vi "PicoScope Test.vi"(2 "WFD-Ref Ch-B":refnum<vi>, 3 "WFD-Ref Ch-A":refnum<vi>, 8 "Acquisition Settings":T3={"preTriggerSamples"=0, "postTriggerSamples"=1000, "timebase"=127, "Down-Sample Mode"=0, "Down Sample Ratio"=1, "Oversample"=0} {"Down Sample Ratio" min=1 step=1; "Down-Sample Mode" items=["None"=0, "Aggregate"=1, "Decimate"=2, "Average"=4]; "postTriggerSamples" max=10000 step=100}, 9 "Trigger Settings":T4={"Trigger Enabled"=FALSE, "Trigger Source"=enum."Channel A", "Trigger Threshold (Volts)"=0.0, "Trigger Direction"=2, "Trigger Delay (samples)"=0, "Auto Trigger Time (ms)"=1000} {"Trigger Direction" items=["Rising"=2, "Falling"=3]}, 10 "Channel B Settings":T1={"Enabled"=TRUE, "Coupling"=1, "Range"=6, "Analogue Offset"=0.0} {"Range" items=["20 mV"=1, "50 mV"=2, "100 mV"=3, "200 mV"=4, "500 mV"=5, "1 V"=6, "2 V"=7, "5 V"=8, "10 V"=9, "20 V"=10]; "Coupling" items=["AC", "DC"]}, 11 "Channel A Settings":T1={"Enabled"=TRUE, "Coupling"=1, "Range"=6, "Analogue Offset"=0.0} {"Range" items=["20 mV"=1, "50 mV"=2, "100 mV"=3, "200 mV"=4, "500 mV"=5, "1 V"=6, "2 V"=7, "5 V"=8, "10 V"=9, "20 V"=10]; "Coupling" items=["AC", "DC"]}) -> (0 "error out":errorcluster, 5 "Properties Panel":T2 {"Max Total Capture Time Available (sec)" format="%.3p"; "Sample Frequency" format="%.3p"; "Sample Internal" format="%.3p"; "Max Samples Available" format="%.3p"; "Total Capture Time (sec)" format="%.3p"})   [LabVIEW 2018]
panel:
  out "Channel B":cluster{i32, "Sample Internal":sgl, dbl[]}(graph)
  out "Peak To Peak":dbl
  out "Channel A":cluster{i32, "Sample Internal":sgl, dbl[]}(graph)
  out "Serial":string
  out "PicoScope Type":string
  # "Dev Info"
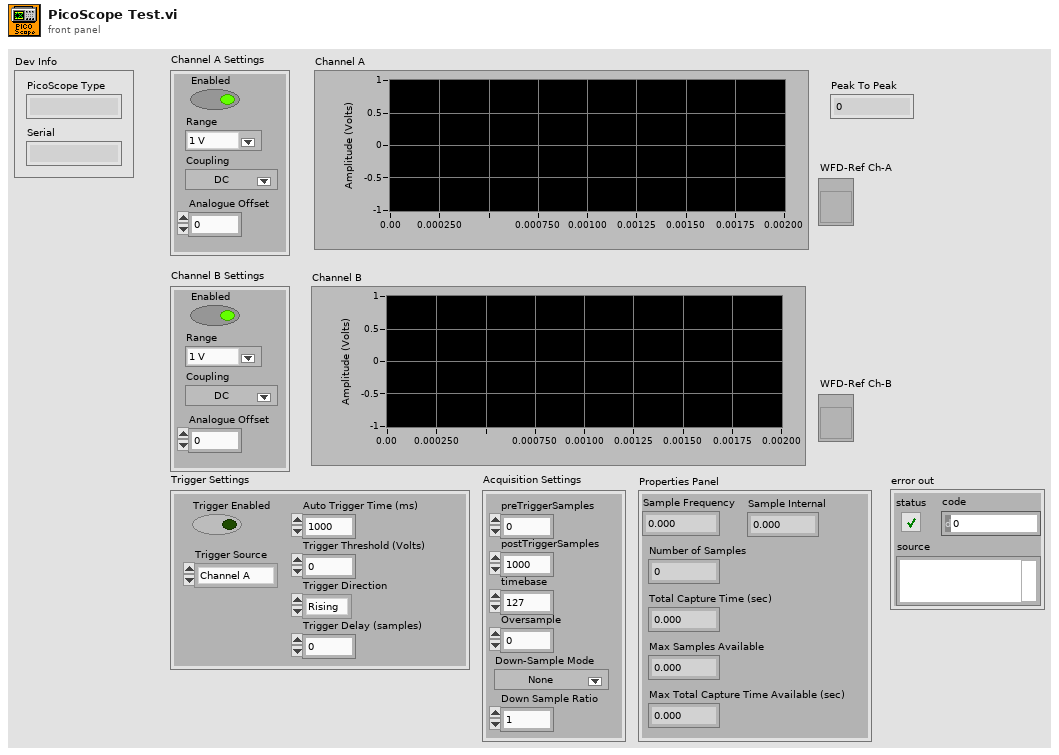
[diagram p1: front panel]
types:
  T1 = cluster{"Enabled":bool, "Coupling":i16, "Range":u16, "Analogue Offset":sgl}
  T2 = cluster{"Sample Frequency":sgl, "Sample Internal":sgl, "Max Samples Available":i32, "Number of Samples":u32, "Total Capture Time (sec) ":sgl, "Max Total Capture Time Available (sec)":sgl}
  T3 = cluster{"preTriggerSamples":u32, "postTriggerSamples":u32, "timebase":u32, "Down-Sample Mode":i32, "Down Sample Ratio":u32, "Oversample":i16}
  T4 = cluster{"Trigger Enabled":bool, "Trigger Source":enum16{"Channel A", "Channel B", "Channel C", "Channel D", "Ext."}, "Trigger Threshold (Volts)":dbl, "Trigger Direction":u16, "Trigger Delay (samples)":u32, "Auto Trigger Time (ms)":i16}
  T5 = cluster{"Driver Version":string, "USB Version":string, "Hardware":string, "Variant":string, "Batch and Serial":string, "Cal Date":string, "Kernel Version":string, "Digital HW Version":string, "Analogue HW Version":string, "Firmware 1":string, "Firmware 2":string, "MSO":bool, "Number of Channels":i16}
  T6 = cluster{"Channel D Buffer":i16[], "Channel C Buffer":i16[], "Channel B Buffer":i16[], "Channel A Buffer":i16[], "Port 0  Buffer ":i16[], "Port 1 Buffer ":i16[]}
  T7 = cluster{i32, "Sample Internal":sgl, "Data (Volts)":dbl[]}
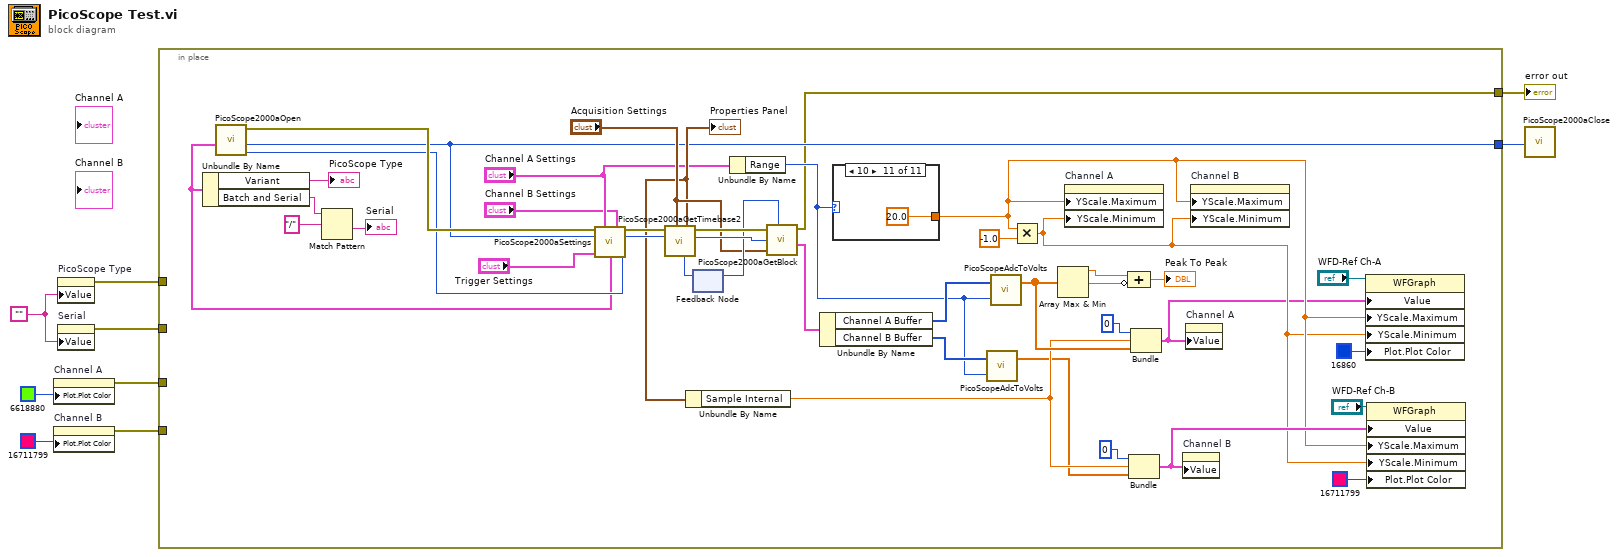
[diagram p0: block diagram]
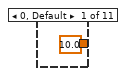
[diagram p2: hidden frame]
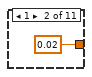
[diagram p3: hidden frame]
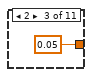
[diagram p4: hidden frame]
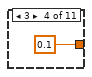
[diagram p5: hidden frame]
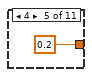
[diagram p6: hidden frame]
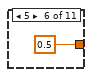
[diagram p7: hidden frame]
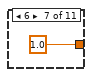
[diagram p8: hidden frame]
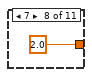
[diagram p9: hidden frame]
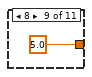
[diagram p10: hidden frame]
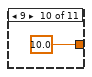
[diagram p11: hidden frame]
diagram:
  w7 = ""
  n1 = property on="Channel A" class="WFGraph (strict)"("Plot.Plot Color"=u32 6618880) -> (error out=w4:errorcluster)  [unwired: 2 in, 1 out]
  n2 = property on="Channel B" class="WFGraph (strict)"("Plot.Plot Color"=u32 16711799) -> (error out=w3:errorcluster)  [unwired: 2 in, 1 out]
  n3 = property on="PicoScope Type" class="Str"("Value"=w7) -> (error out=w9:errorcluster)  [unwired: 2 in, 1 out]
  n4 = property on="Serial" class="Str"("Value"=w7) -> (error out=w8:errorcluster)  [unwired: 2 in, 1 out]
  n5 = in-place {
    in-place-border: w9 -> [_]
    in-place-border: w8 -> [_]
    in-place-border: w4 -> [_]
    in-place-border: w3 -> [_]
    in-place-border: [w14] -> w2
    in-place-border: [w13] -> w1
    n6 = call "PicoScope2000aOpen.vi"() -> ("Max Adc value"=w45:i16, "handle"=w14:i16, "error out"=w46:errorcluster, "Device Info"=w44:T5)  [unwired: 4 in]
    n7 = Unbundle By Name(w44) -> ("Variant"=→"PicoScope Type":string, "Batch and Serial"=w49:string)
    n8 = Match Pattern(string=w49, regular expression="/") -> (after substring=→"Serial":string)  [unwired: 1 in, 3 out]
    n9 = call "PicoScope2000aSettings.vi"("error in"=w46, "Channel A Settings"="Channel A Settings", "Channel B Settings"="Channel B Settings", "handle in"=w14, "Trigger Settings"="Trigger Settings", "Device Info"=w44, "Max_adc"=w45) -> ("error out"=w42:errorcluster, "handle out"=w41:i16)  [unwired: 6 in, 1 out]
    n10 = feedback #1() -> (w37:u32)  [unwired: 1 in]
    n11 = call "PicoScope2000aGetTimebase2.vi"("Number of Samples"=w37, "Acquisition Settings"="Acquisition Settings", "handle in"=w41, "error in (no error)"=w42) -> ("handle out"=w39:i16, "error out"=w40:errorcluster, "Properties Panel"=w33:T2)  [unwired: 5 in]
    "Properties Panel" <- w33
    n12 = Unbundle By Name(w33) -> ("Sample Internal"=w21:sgl)
    n13 = Unbundle By Name("Channel A Settings") -> ("Range"=w23:u16)
    n14 = call "PicoScope2000aGetBlock.vi"("error in"=w40, "handle in"=w39, "Acquisition Settings"="Acquisition Settings") -> ("noOfSamples"=w38:u32, "error out"=w13:errorcluster, "Buffers (Max or non-aggregated)"=w35:T6)  [unwired: 2 in, 3 out]
    n15 = feedback-in #1(w38) -> ()
    n16 = Unbundle By Name(w35) -> ("Channel A Buffer"=w32:i16[], "Channel B Buffer"=w24:i16[])
    n17 = case shown="10" w23 {
      tunnel: [10.0 0.02 0.05 0.1 0.2 0.5 1.0 2.0 5.0 10.0 20.0] -> w16
      frame 0, Default {
      }
      frame 1 {
      }
      frame 2 {
      }
      frame 3 {
      }
      frame 4 {
      }
      frame 5 {
      }
      frame 6 {
      }
      frame 7 {
      }
      frame 8 {
      }
      frame 9 {
      }
      frame 10 {
      }
    }
    n18 = call "PicoScopeAdcToVolts.vi"("Range Index"=w23, "Data"=w24) -> ("Data (Volts)"=w20:dbl[])  [unwired: 1 in]
    n19 = call "PicoScopeAdcToVolts.vi"("Range Index"=w23, "Data"=w32) -> ("Data (Volts)"=w30:dbl[])  [unwired: 1 in]
    n20 = Multiply(x=w16, y=-1.0) -> (x*y=w15:dbl)
    n21 = Array Max & Min(array=w30) -> (max value=w28:dbl, min value=w26:dbl)  [unwired: 2 out]
    n22 = property on="Channel A" class="WFGraph (strict)"("YScale.Maximum"=w16, "YScale.Minimum"=w15) -> ()  [unwired: 2 in, 2 out]
    n23 = Compound Arithmetic op=ADD(w28, invert w26) -> (→"Peak To Peak":dbl)
    n24 = Bundle(0, "Sample Internal"=w21, "Data (Volts)"=w20) -> (w18:T7)  [unwired: 1 in]
    n25 = Bundle(0, "Sample Internal"=w21, "Data (Volts)"=w30) -> (w12:T7)  [unwired: 1 in]
    n26 = property on="Channel B" class="WFGraph (strict)"("Value"=w18) -> ()  [unwired: 2 in, 2 out]
    n27 = property on="Channel A" class="WFGraph (strict)"("Value"=w12) -> ()  [unwired: 2 in, 2 out]
    n28 = property on="Channel B" class="WFGraph (strict)"("YScale.Maximum"=w16, "YScale.Minimum"=w15) -> ()  [unwired: 2 in, 2 out]
    n29 = property class="WFGraph"(reference="WFD-Ref Ch-A", "Value"=w12, "YScale.Maximum"=w16, "YScale.Minimum"=w15, "Plot.Plot Color"=u32 16860) -> ()  [unwired: 1 in, 2 out]
    n30 = property class="WFGraph"(reference="WFD-Ref Ch-B", "Value"=w18, "YScale.Maximum"=w16, "YScale.Minimum"=w15, "Plot.Plot Color"=u32 16711799) -> ()  [unwired: 1 in, 2 out]
  }
  "error out" <- w1
  n31 = call "PicoScope2000aClose.vi"("handle"=w2) -> ()
